vi "10-2.vi"() -> ()   [LabVIEW 2019, in "10.lvlib"]
uses:
  10.lvlib
  <vilib>/Analysis/NI_AALBase.lvlib
panel:
  out "Middle Score":u64
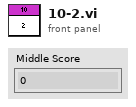
[diagram p1: front panel]
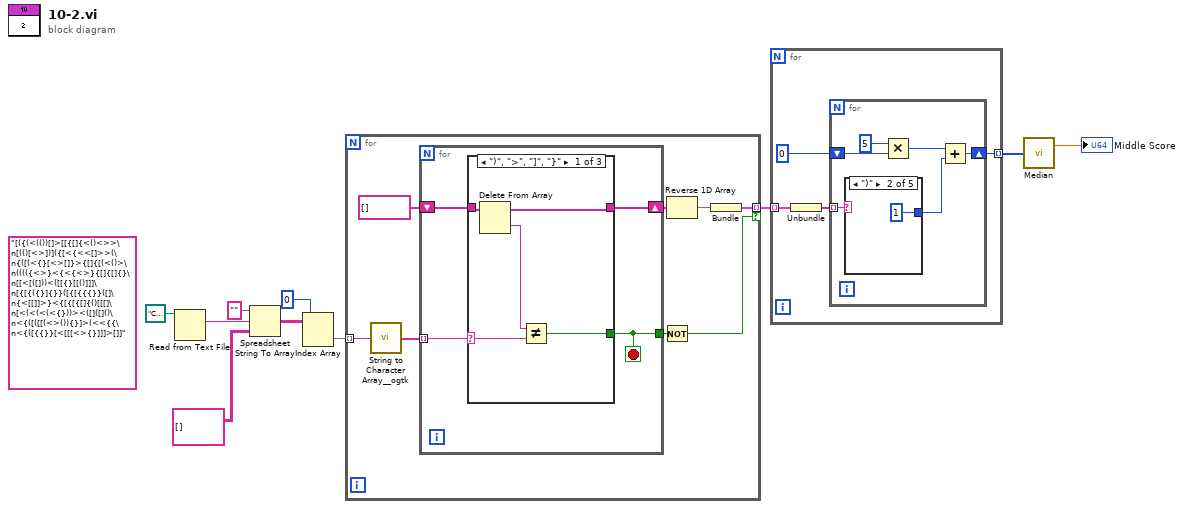
[diagram p0: block diagram]
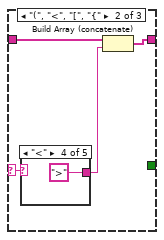
[diagram p2: hidden frame]
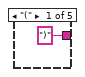
[diagram p3: hidden frame]
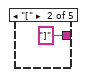
[diagram p4: hidden frame]
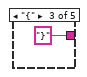
[diagram p5: hidden frame]
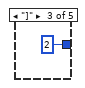
[diagram p9: hidden frame]
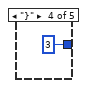
[diagram p10: hidden frame]
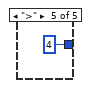
[diagram p11: hidden frame]
diagram:
  (unwired) "[({(<(())[]>[[{[]{<()<>>\n[(()[<>])]({[<{<<[]>>(\n{([(<{}[<>[]}>{[]{[(<()>\n(((({<>}<{<{<>}{[]{[]{}\n[[<[([]))<([[{}[[()]]]\n[{[{({}]{}}([{[{{{}}([]\n{<[[]]>}<{[{[{[]{()[[[]\n[<(<(<(<{}))><([]([]()\n<{([([[(<>()){}]>(<<{{\n<{([{{}}[<[[[<>{}]]]>[]]"
  n1 = Read from Text File(file (use dialog)=path "C:/Users/craig.walker/Documents/GitHub/lv2019-Advent-of-Code-2021/10/input.txt") -> (text=w3:string)  [unwired: 3 in, 3 out]
  n2 = Spreadsheet String To Array(format string="", spreadsheet string=w3, array type (2D Dbl)=string[][] []) -> (array=w7:string[][])  [unwired: 1 in]
  n3 = Index Array(array=w7, index (col)=0 ("disabled index (col)")) -> (element=w8:string[])  [unwired: 1 in]
  n4 = for {
    tunnel: w8 -> [w18] mode=indexing
    tunnel: [w11] -> w4 mode=indexing if=w13
    n5 = call <userlib>:"String to Character Array__ogtk.vi"("Input String"=w18) -> ("Character Array"=w17:string[])
    n6 = for {
      tunnel: w17 -> [w22] mode=indexing
      tunnel: [w21] -> w16
      shift-right: [w20] -> w14
      shift-left: string[] [] -> [w19]
      stop <- w21 stop-if-true
      n7 = case shown="\")\", \">\", \"]\", \"}\"" w22 {
        selector: w22 -> [w23 w29 _]
        tunnel: [w25 _ _] -> w21
        tunnel: [w26 w31 w36] -> w20
        tunnel: w19 -> [w27 w30 w36]
        frame ")", ">", "]", "}" {
          n8 = Delete From Array(array=w27) -> (deleted portion=w24:string, array with subset deleted=w26:string[])  [unwired: 2 in]
          n9 = Not Equal?(x=w24, y=w23) -> (x != y?=w25:bool)
        }
        frame "(", "<", "[", "{" {
          n10 = case shown="\"<\"" w29 {
            tunnel: [")" ("]") "]" ("]") "}" ("]") ">" ("]") _] -> w28
            frame "(" {
            }
            frame "[" {
            }
            frame "{" {
            }
            frame "<" {
            }
            frame Default {
            }
          }
          n11 = Build Array (concatenate)(w30, w28) -> (w31:string[])
        }
        frame Default {
        }
      }
    }
    n12 = Not(x=w16) -> (.not. x?=w13:bool)
    n13 = Reverse 1D Array(array=w14) -> (reversed array=w12:string[])
    n14 = Bundle(w12) -> (w11:cluster{string[]})  [unwired: 1 in]
  }
  n15 = for {
    tunnel: w4 -> [w40] mode=indexing
    tunnel: [w39] -> w2 mode=indexing
    n16 = Unbundle(w40) -> (w38:string[])
    n17 = for {
      tunnel: w38 -> [w46] mode=indexing
      shift-right: [w42] -> w39
      shift-left: u64 0 ("disabled index (col)") -> [w41]
      n18 = case shown="\")\"" w46 {
        tunnel: [_ u64 1 ("disabled index (col)") u64 2 ("disabled index (col)") u64 3 ("disabled index (col)") u64 4 ("disabled index (col)")] -> w43
        frame Default {
        }
        frame ")" {
        }
        frame "]" {
        }
        frame "}" {
        }
        frame ">" {
        }
      }
      n19 = Multiply(x=u64 5, y=w41) -> (x*y=w45:u64)
      n20 = Add(x=w45, y=w43) -> (x+y=w42:u64)
    }
  }
  n21 = call <vilib>:"Median.vi"("X"=w2) -> ("median"=→"Middle Score":dbl)  [unwired: 1 out]
